vi "Parse DB - 1553 - Get RT Config.vi"(0 "channel config handle":u32, 11 "error in (no error)":errorcluster) -> (4 "channel config handle out":u32, 8 "RT_Messages":T1[](array[typedef]), 15 "error out":errorcluster)   [LabVIEW 2013]
uses:
  Controls/1553_RT_Message.ctl
  Controls/664 -Param.ctl
  AIT 664 Custom Device.lvlib
  <userlib>/MIL-STD-1553/Owl1553.lvlib
panel:
  out "RT Tx Array":bool[][](array[boolean])
  out "RT Rx Array":bool[][](array[boolean])
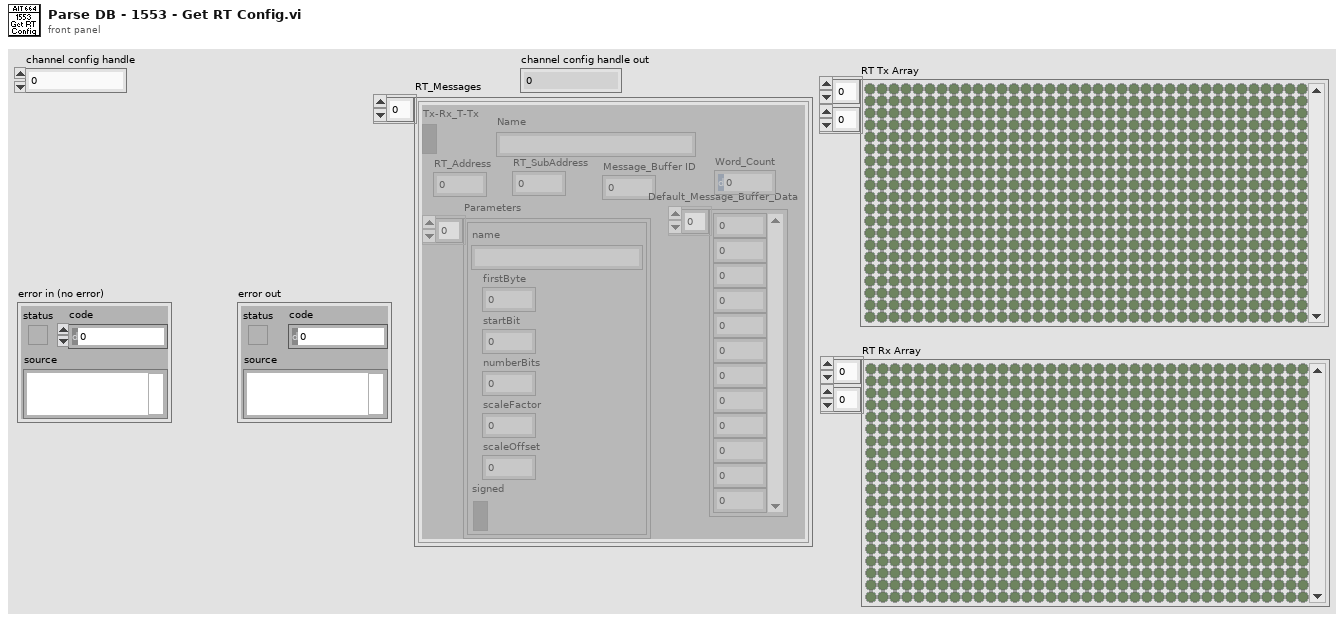
[diagram p1: front panel]
types:
  T1 = typedef "AIT 664 Custom Device.lvlib/1553_RT_Message.ctl" = cluster{"RT_Address":u8, "RT_SubAddress":u8, "Tx-Rx_T-Tx":bool, "Parameters":T2[], "Message_Buffer ID":u16, "Default_Message_Buffer_Data":u16[], "Word_Count":u8, "Name":string}
  T2 = typedef "AIT 664 Custom Device.lvlib/664 -Param.ctl" = cluster{"name":string, "firstByte":i32, "startBit":i32, "numberBits":i32, "scaleFactor":dbl, "scaleOffset":dbl, "signed":bool}
  T3 = enum16{"OWL1553_RECEIVE_TRANSFER", "OWL1553_TRANSMIT_TRANSFER"}
  T4 = enum16{"OWL_1553_MILBUS_CHANNEL_PRIMARY", "OWL_1553_MILBUS_CHANNEL_SECONDARY"}
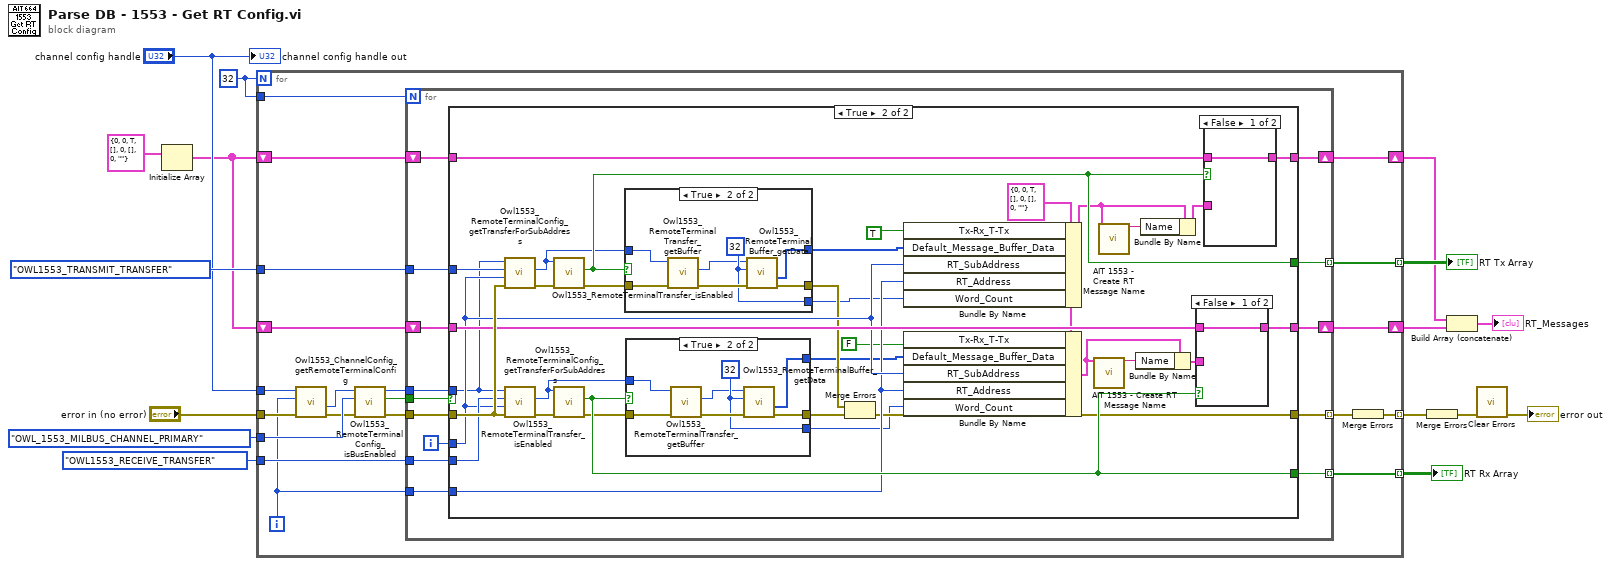
[diagram p0: block diagram]
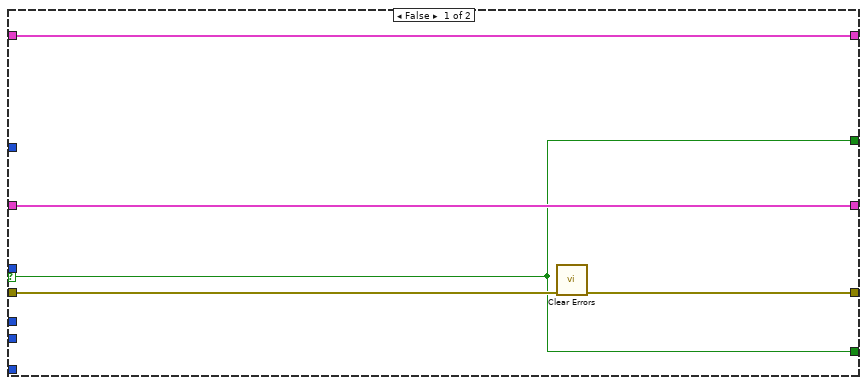
[diagram p2: hidden frame]
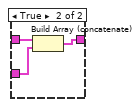
[diagram p3: hidden frame]
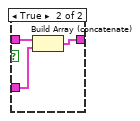
[diagram p5: hidden frame]
diagram:
  w10 = 32
  n1 = Initialize Array(T1 {"RT_Address"=0, "RT_SubAddress"=0, "Tx-Rx_T-Tx"=TRUE, "Parameters"=[], "Message_Buffer ID"=0, "Default_Message_Buffer_Data"=[], "Word_Count"=0, "Name"=""} ("RT_Message")) -> (w1:T1[])  [unwired: 1 in]
  n2 = for {
    N: w10 -> [_]
    tunnel: T4."OWL_1553_MILBUS_CHANNEL_PRIMARY" ("milbus") -> [w35]
    tunnel: [w17] -> w14 mode=indexing
    tunnel: "channel config handle" -> [w36]
    tunnel: "error in (no error)" -> [w32]
    tunnel: w10 -> [w29]
    tunnel: [w28] -> w7 mode=indexing
    tunnel: T3."OWL1553_TRANSMIT_TRANSFER" ("direction") -> [w26]
    tunnel: T3."OWL1553_RECEIVE_TRANSFER" ("direction") -> [w25]
    tunnel: [w24] -> w8 mode=indexing
    shift-right: [w23] -> w4
    shift-left: w1 -> [w22]
    shift-right: [w20] -> w5
    shift-left: w1 -> [w21]
    i -> [w19]
    n3 = call <userlib>:"Owl1553_ChannelConfig_getRemoteTerminalConfig.vi"("error in (no error)"=w32, "remote terminal"=w19, "channel config handle"=w36) -> ("error out"=w34:errorcluster, "remote terminal config handle"=w33:u64)  [unwired: 5 in, 2 out]
    n4 = call <userlib>:"Owl1553_RemoteTerminalConfig_isBusEnabled.vi"("error in (no error)"=w34, "milbus"=w35, "remote terminal config handle"=w33) -> ("error out"=w31:errorcluster, "is enabled"=w30:bool, "remote terminal config handle"=w27:u64)  [unwired: 6 in]
    n5 = for {
      N: w29 -> [_]
      tunnel: [w47] -> w18 mode=indexing
      tunnel: w31 -> [w50]
      tunnel: w30 -> [w49]
      tunnel: [w48] -> w28 mode=indexing
      tunnel: w27 -> [w46]
      tunnel: w26 -> [w45]
      tunnel: w25 -> [w44]
      tunnel: [w43] -> w24 mode=indexing
      shift-right: [w42] -> w23
      shift-left: w22 -> [w41]
      shift-right: [w39] -> w20
      shift-left: w21 -> [w40]
      tunnel: w19 -> [w37]
      i -> [w38]
      n6 = case shown="True" w49 {
        selector: w49 -> [w51 _]
        tunnel: [w54 w71] -> w47
        tunnel: w50 -> [w55 w86]
        tunnel: [w51 w80] -> w48
        tunnel: w46 -> [_ w75]
        tunnel: w38 -> [_ w76]
        tunnel: w45 -> [_ w89]
        tunnel: w44 -> [_ w77]
        tunnel: [w51 w79] -> w43
        tunnel: [w53 w84] -> w42
        tunnel: w41 -> [w53 w85]
        tunnel: w40 -> [w52 w83]
        tunnel: [w52 w82] -> w39
        tunnel: w37 -> [_ w74]
        frame False {
          n7 = call <vilib>:"Clear Errors.vi"("error in (no error)"=w55) -> ("error out"=w54:errorcluster)  [unwired: 6 in]
        }
        frame True {
          w68 = T1 {"RT_Address"=0, "RT_SubAddress"=0, "Tx-Rx_T-Tx"=TRUE, "Parameters"=[], "Message_Buffer ID"=0, "Default_Message_Buffer_Data"=[], "Word_Count"=0, "Name"=""} ("RT_Message")
          n8 = call <userlib>:"Owl1553_RemoteTerminalConfig_getTransferForSubAddress.vi"("error in (no error)"=w86, "sub address"=w76, "direction"=w89, "remote terminal config handle"=w75) -> ("error out"=w88:errorcluster, "transfer handle"=w62:u64)  [unwired: 5 in, 1 out]
          n9 = call <userlib>:"Owl1553_RemoteTerminalConfig_getTransferForSubAddress.vi"("error in (no error)"=w86, "sub address"=w76, "direction"=w77, "remote terminal config handle"=w75) -> ("error out"=w87:errorcluster, "transfer handle"=w63:u64)  [unwired: 5 in, 1 out]
          n10 = call <userlib>:"Owl1553_RemoteTerminalTransfer_isEnabled.vi"("error in (no error)"=w88, "remote terminal transfer handle"=w62) -> ("error out"=w81:errorcluster, "is enabled"=w80:bool)  [unwired: 7 in, 1 out]
          n11 = call <userlib>:"Owl1553_RemoteTerminalTransfer_isEnabled.vi"("error in (no error)"=w87, "remote terminal transfer handle"=w63) -> ("error out"=w78:errorcluster, "is enabled"=w79:bool)  [unwired: 7 in, 1 out]
          n12 = case shown="True" w80 {
            tunnel: w81 -> [w106 w111]
            tunnel: [w106 w113] -> w73
            tunnel: [_ w112] -> w69
            tunnel: [_ w108] -> w65
            tunnel: w62 -> [_ w110]
            frame False {
            }
            frame True {
              w108 = u32 32
              n13 = call <userlib>:"Owl1553_RemoteTerminalTransfer_getBuffer.vi"("error in (no error)"=w111, "remote terminal transfer handle"=w110) -> ("error out"=w109:errorcluster, "buffer"=w107:u64)  [unwired: 7 in, 1 out]
              n14 = call <userlib>:"Owl1553_RemoteTerminalBuffer_getData.vi"("error in (no error)"=w109, "buffer size"=w108, "buffer handle"=w107) -> ("error out"=w113:errorcluster, "data"=w112:u16[])  [unwired: 5 in, 2 out]
            }
          }
          n15 = case shown="True" w79 {
            tunnel: w78 -> [w94 w99]
            tunnel: [w94 w101] -> w72
            tunnel: [_ w95] -> w70
            tunnel: [_ w97] -> w64
            tunnel: w63 -> [_ w100]
            frame False {
            }
            frame True {
              w97 = u32 32
              n16 = call <userlib>:"Owl1553_RemoteTerminalTransfer_getBuffer.vi"("error in (no error)"=w99, "remote terminal transfer handle"=w100) -> ("error out"=w98:errorcluster, "buffer"=w96:u64)  [unwired: 7 in, 1 out]
              n17 = call <userlib>:"Owl1553_RemoteTerminalBuffer_getData.vi"("error in (no error)"=w98, "buffer size"=w97, "buffer handle"=w96) -> ("error out"=w101:errorcluster, "data"=w95:u16[])  [unwired: 5 in, 2 out]
            }
          }
          n18 = Merge Errors(w73, w72) -> (w71:errorcluster)
          n19 = Bundle By Name(cluster=w68, "Tx-Rx_T-Tx"=TRUE ("Tx-Rx (T=Tx)"), "Default_Message_Buffer_Data"=w69, "RT_SubAddress"=w76, "RT_Address"=w74, "Word_Count"=w65) -> (w61:T1)
          n20 = Bundle By Name(cluster=w68, "Tx-Rx_T-Tx"=FALSE ("Tx-Rx (T=Tx)"), "Default_Message_Buffer_Data"=w70, "RT_SubAddress"=w76, "RT_Address"=w74, "Word_Count"=w64) -> (w57:T1)
          n21 = call "AIT 1553 - Create RT Message Name.vi"("RT_Message"=w57) -> ("Message Name"=w58:string)  [unwired: 13 in, 1 out]
          n22 = call "AIT 1553 - Create RT Message Name.vi"("RT_Message"=w61) -> ("Message Name"=w59:string)  [unwired: 13 in, 1 out]
          n23 = Bundle By Name(cluster=w57, "Name"=w58) -> (w56:T1)
          n24 = Bundle By Name(cluster=w61, "Name"=w59) -> (w60:T1)
          n25 = case shown="False" w79 {
            tunnel: w83 -> [w90 w93]
            tunnel: w56 -> [_ w92]
            tunnel: [w90 w91] -> w82
            frame False {
            }
            frame True {
              n26 = Build Array (concatenate)(w93, w92) -> (w91:T1[])
            }
          }
          n27 = case shown="False" w80 {
            tunnel: w85 -> [w102 w105]
            tunnel: w60 -> [_ w104]
            tunnel: [w102 w103] -> w84
            frame False {
            }
            frame True {
              n28 = Build Array (concatenate)(w105, w104) -> (w103:T1[])
            }
          }
        }
      }
    }
    n29 = Merge Errors(w18) -> (w17:errorcluster)
  }
  "RT Tx Array" <- w7
  "RT Rx Array" <- w8
  n30 = Merge Errors(w14) -> (w9:errorcluster)
  n31 = Build Array (concatenate)(w4, w5) -> (→"RT_Messages":T1[])
  n32 = call <vilib>:"Clear Errors.vi"("error in (no error)"=w9) -> ("error out"=→"error out":errorcluster)  [unwired: 6 in]
  "channel config handle out" <- "channel config handle"
